vi "remove_edge.vi"(8 "error in (no error)":errorcluster, 11 "Edge in":refnum<class "Edge.lvclass">) -> (0 "error out":errorcluster, 3 "Edge out":refnum<class "Edge.lvclass">)   [LabVIEW 2020]
uses:
  Edge.lvclass/Edge.ctl
  Edge.lvclass
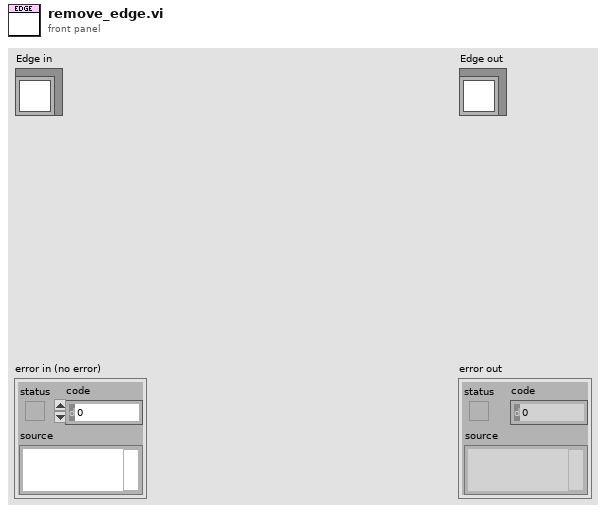
[diagram p1: front panel]
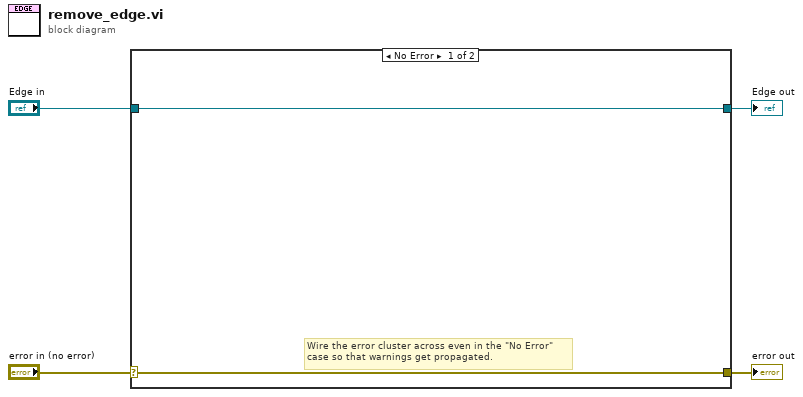
[diagram p0: block diagram]
diagram:
  n1 = case shown="No Error" "error in (no error)" {
    selector: "error in (no error)" -> [w5 w8]
    tunnel: [w5 w8] -> w3
    tunnel: [w6 w7] -> w1
    tunnel: "Edge in" -> [w6 w7]
    frame No Error {
      # "Wire the error cluster across even in the \"No Error\"\ncase so that warnings get propagated."
    }
    frame Error {
    }
  }
  "error out" <- w3
  "Edge out" <- w1
